vi "Autonomous Independent.vi"   [LabVIEW 2016]
doc: "This VI is called when autonomous begins, and will automatically be terminated when autonomous ends. You can carry out timed or sensor driven robot movement independently without needing to return to the caller."
uses:
  <vilib>/Rock Robotics/WPI/Utilities/WPI_GetSetVariantRefNum.vi
  <vilib>/Rock Robotics/Network Tables/NT Read String.vi
  Robot Global Data.vi
  <vilib>/Rock Robotics/Network Tables/NT Write Numeric Array.vi
  <vilib>/Rock Robotics/Network Tables/NT Read Number.vi
panel:
  # "Be sure to right-click and choose Data Operations>>Make Current Value default if you want to save the array values with the VI"
types:
  T1 = typedef "WPI_JoystickDevRef.ctl" = cluster{"Device":T2}
  T2 = typedef "WPI_JoystickDeviceEnum.ctl" = enum16{"USB 0", "USB 1", "USB 2", "USB 3", "USB 4", "USB 5"}
  T3 = enum16{"Front Left", "Front Right", "Back Left", "Back Right"}
  T4 = cluster{"Yaw":dbl, "Roll":dbl, "Pitch":dbl, "Heading":dbl, "Fused Heading":dbl}
  T5 = typedef "WPI_MotorControlDeviceRef.ctl" = cluster{"DeviceStatus":errorcluster, "Type":T6, "PWM":cluster{"PWM Channel":T7, "DeadBand":T8}, "CAN":cluster{"Device Number":u8, "SetOutput VI Ref":variant, "GetOutput VI Ref":variant, "Enable VI Ref":variant, "Disable VI Ref":variant, "Data":variant}, "Invert":bool}
  T6 = typedef "WPI_MotorControlType.ctl" = enum16{"PWM", "CAN"}
  T7 = typedef "FPGA_DIOPWMChannel.ctl" = enum8{"PWM 0", "PWM 1", "PWM 2", "PWM 3", "PWM 4", "PWM 5", "PWM 6", "PWM 7", "PWM 8", "PWM 9", "PWM MXP 0", "PWM MXP 1", "PWM MXP 2", "PWM MXP 3", "PWM MXP 4", "PWM MXP 5", "PWM MXP 6", "PWM MXP 7", "PWM MXP 8", "PWM MXP 9", "Invalid"}
  T8 = typedef "WPI_PWMDeadband.ctl" = cluster{"Name":string, "maxPositivePwm":i32, "minPositivePwm":i32, "centerPwm":i32, "maxNegativePwm":i32, "minNegativePwm":i32, "angularRange":u16}
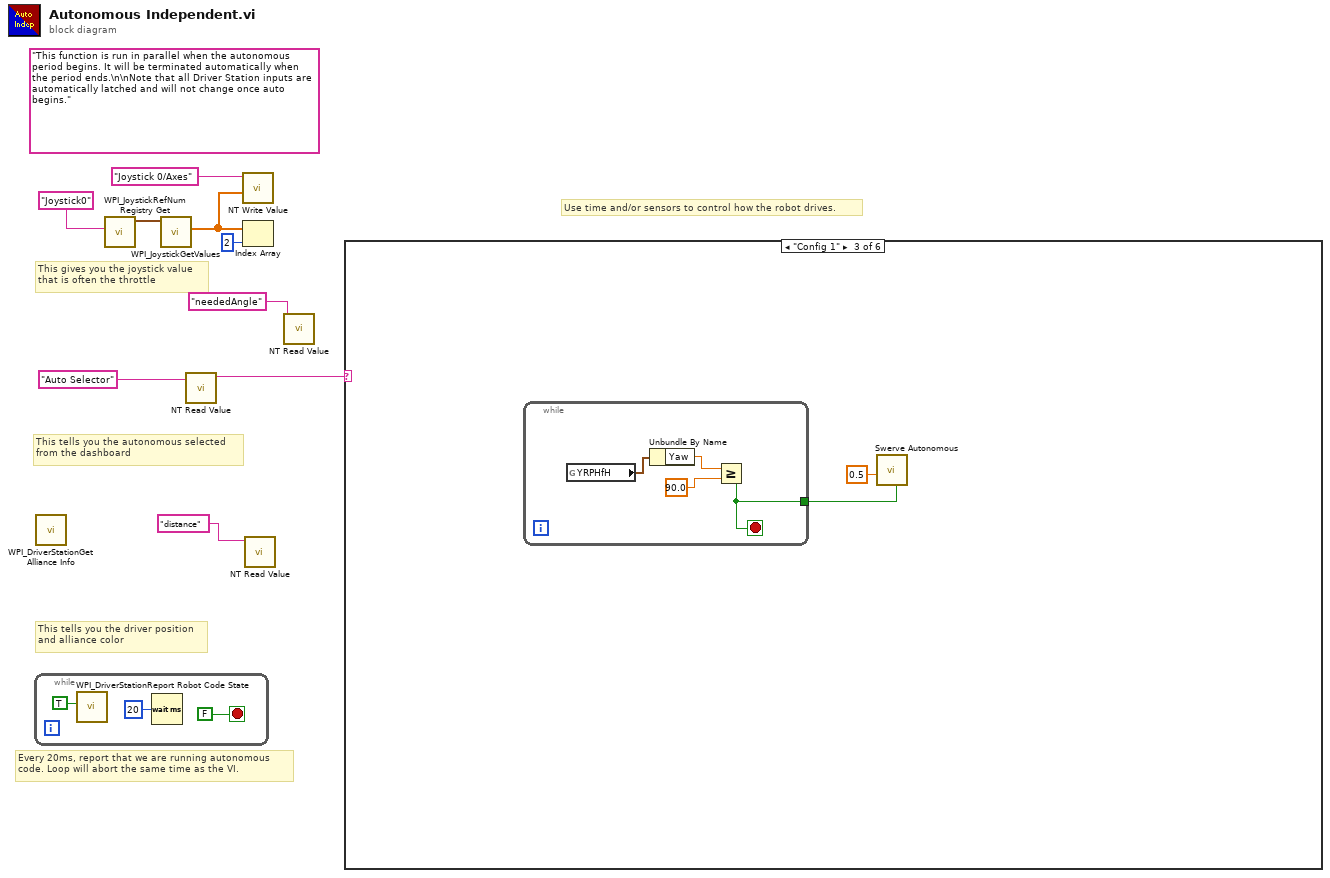
[diagram p0: block diagram]
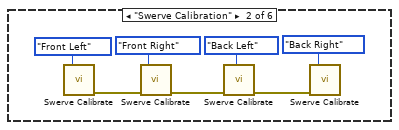
[diagram p3: hidden frame]
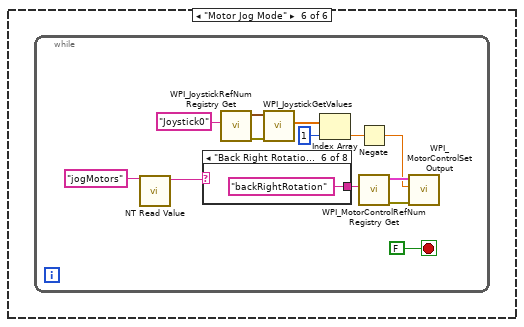
[diagram p6: hidden frame]
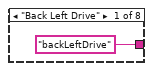
[diagram p7: hidden frame]
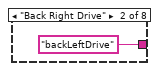
[diagram p8: hidden frame]
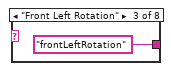
[diagram p9: hidden frame]
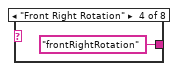
[diagram p10: hidden frame]
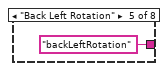
[diagram p11: hidden frame]
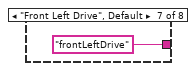
[diagram p12: hidden frame]
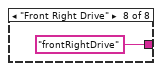
[diagram p13: hidden frame]
diagram:
  (unwired) "This function is run in parallel when the autonomous period begins. It will be terminated automatically when the period ends.\n\nNote that all Driver Station inputs are automatically latched and will not change once auto begins."
  # "This tells you the autonomous selected\nfrom the dashboard"
  # "Every 20ms, report that we are running autonomous\ncode. Loop will abort the same time as the VI."
  # "This gives you the joystick value\nthat is often the throttle"
  # "Use time and/or sensors to control how the robot drives."
  # "This tells you the driver position\nand alliance color"
  n1 = while {
    stop <- FALSE stop-if-true
    n2 = call <vilib>:"WPI_DriverStationReport Robot Code State.vi"("Autonomous"=TRUE) -> ()  [unwired: 10 in, 1 out]
    n3 = Wait (ms)(milliseconds to wait=u32 20) -> ()  [unwired: 1 out]
  }
  n4 = call <vilib>:"WPI_DriverStationGet Alliance Info.vi"() -> ()  [unwired: 12 out]
  n5 = call <vilib>:"WPI_JoystickRefNum Registry Get.vi"("refnum name"="Joystick0") -> ("JoystickDevRef"=w8:T1)  [unwired: 1 in, 9 out]
  n6 = call <vilib>:"WPI_JoystickGetValues.vi"("JoystickDevRef"=w8) -> ("Axes"=w4:dbl[])  [unwired: 6 in, 4 out]
  n7 = call-poly <vilib>:"NT Read Value.vi"("Name"="Auto Selector") -> ("String"=w5:string)  [unwired: 9 in, 1 out]
  n8 = call-poly <vilib>:"NT Write Value.vi"("Numeric Array"=w4, "Name"="Joystick 0/Axes") -> ()  [unwired: 9 in, 1 out]
  n9 = Index Array(array=w4, index=2) -> ()  [unwired: 1 out]
  n10 = call-poly <vilib>:"NT Read Value.vi"("Name"="distance") -> ()  [unwired: 9 in, 2 out]
  n11 = call-poly <vilib>:"NT Read Value.vi"("Name"="neededAngle") -> ()  [unwired: 9 in, 2 out]
  n12 = case shown="\"Config 1\"" w5 {
    frame Default {
      # "You can put your main auto here, or you can right-click on the case and make any\nother frame be the default case."
      # "This is the frame that will execute if no selection is made, or if it is not recognized"
    }
    frame "Swerve Calibration" {
      n13 = call "Swerve Calibrate.vi"("Wheel Corner"=T3."Front Left") -> ("error out"=w15:errorcluster)  [unwired: 10 in]
      n14 = call "Swerve Calibrate.vi"("error in (no error)"=w15, "Wheel Corner"=T3."Front Right") -> ("error out"=w14:errorcluster)  [unwired: 9 in]
      n15 = call "Swerve Calibrate.vi"("error in (no error)"=w14, "Wheel Corner"=T3."Back Left") -> ("error out"=w13:errorcluster)  [unwired: 9 in]
      n16 = call "Swerve Calibrate.vi"("error in (no error)"=w13, "Wheel Corner"=T3."Back Right") -> ()  [unwired: 9 in, 1 out]
    }
    frame "Config 1" {
      n17 = while {
        tunnel: [w22] -> w21
        stop <- w22 stop-if-true
        n18 = global read "Robot Global Data.vi" "YRPHfH"() -> (w25:T4)
        n19 = Unbundle By Name(w25) -> ("Yaw"=w24:dbl)
        n20 = Greater Or Equal?(x=w24, y=90.0) -> (x >= y?=w22:bool)
      }
      n21 = call "Swerve Autonomous.vi"("Alternate Stop"=w21, "Z"=0.5) -> ()  [unwired: 9 in, 1 out]
    }
    frame "Config 2" {
    }
    frame "Config 3" {
    }
    frame "Motor Jog Mode" {
      n22 = while {
        stop <- FALSE stop-if-true
        n23 = call-poly <vilib>:"NT Read Value.vi"("Name"="jogMotors") -> ("String"=w29:string)  [unwired: 9 in, 1 out]
        n24 = case shown="\"Back Right Rotation\"" w29 {
          tunnel: ["backLeftDrive" ("refnum name") "backLeftDrive" ("refnum name") "frontLeftRotation" ("refnum name") "frontRightRotation" ("refnum name") "backLeftRotation" ("refnum name") "backRightRotation" ("refnum name") "frontLeftDrive" ("refnum name") "frontRightDrive" ("refnum name")] -> w27
          frame "Back Left Drive" {
          }
          frame "Back Right Drive" {
          }
          frame "Front Left Rotation" {
          }
          frame "Front Right Rotation" {
          }
          frame "Back Left Rotation" {
          }
          frame "Back Right Rotation" {
          }
          frame "Front Left Drive", Default {
          }
          frame "Front Right Drive" {
          }
        }
        n25 = call <vilib>:"WPI_JoystickRefNum Registry Get.vi"("refnum name"="Joystick0") -> ("error out"=w36:errorcluster, "JoystickDevRef"=w37:T1)  [unwired: 1 in, 8 out]
        n26 = call <vilib>:"WPI_JoystickGetValues.vi"("error in (no error)"=w36, "JoystickDevRef"=w37) -> ("Axes"=w35:dbl[])  [unwired: 5 in, 4 out]
        n27 = Index Array(array=w35, index=1) -> (element=w31:dbl)
        n28 = Negate(x=w31) -> (-x=w30:dbl)
        n29 = call <vilib>:"WPI_MotorControlRefNum Registry Get.vi"("refnum name"=w27) -> ("error out"=w33:errorcluster, "MotorControlDevRef"=w32:T5)  [unwired: 9 in]
        n30 = call <vilib>:"WPI_MotorControlSetOutput.vi"("error in (no error)"=w33, "Output"=w30, "MotorControlDevRef"=w32) -> ()  [unwired: 6 in, 3 out]
      }
    }
  }
